vi "Interfaz.vi"() -> ()   [LabVIEW 2018]
uses:
  <vilib>/addons/control/pid/pid.llb/PID EGU to Percentage (DBL).vi
  <vilib>/addons/control/pid/pid.llb/PID Advanced (DBL).vi
  <vilib>/addons/control/pid/NI_PID_pid.lvlib
panel:
  in  "Ring":u16(ring) items=["Principal", "Master", "Slave", "Setting", "Graphics", "Conections"]
  in  "stop":bool
  out "Flux (%)":dbl format="%.2f"
  out "Level (%)":dbl format="%.2f"
  in  "TX Flux":dbl min=0.0 max=0.025
  in  "TX Level":dbl min=0.0 max=0.025
  out "Tab Control":T1(tab)
  out "Level %":dbl
  out "Apertura %":dbl
  out "Flux %":dbl format="%#.1f"
  out "Slide":u8(slide) scale=0.0..100.0
  out "Usuario activo":string
  in  "Please, enterthe  password":string
  in  "Cerrar Sesión":bool
  in  "LSP/ RSP":bool
  out "Fuera De rango":string
  in  "Manual/Auto":bool
  out "Low Limit":bool
  out "High Limit":bool
  in  "Alarm":cluster{dbl, dbl}(slide)={24.183006535947708, 67.3202614379085} scale=0.0..100.0
  in  "SP:":dbl(slide)=54.966887417218544 min=0.0 max=0.0 scale=0.0..100.0
  out "AV:":dbl(slide)=100.0 scale=0.0..100.0
  out "PV:":dbl(slide)=33.01408837398299 scale=0.0..100.0
  in  "MV:":dbl(slide)=100.0 min=0.0 max=100.0 scale=0.0..100.0
  out "RSP:":dbl(slide)=54.966887417218544 min=0.0 max=0.0 scale=0.0..100.0
  out "AV: S":dbl(slide)=100.0 scale=0.0..100.0
  out "Fuera De rango S":string
  in  "Manual/Auto Slave":bool
  out "Low Limit S":bool
  out "High Limit S":bool
  in  "Alarm S":cluster{dbl, dbl}(slide)={24.183006535947708, 67.3202614379085} scale=0.0..100.0
  in  "LSP":dbl(slide)=54.966887417218544 min=0.0 max=0.0 scale=0.0..100.0
  in  "MV: S":dbl(slide)=100.0 scale=-100.0..100.0
  out "PV: S":dbl(slide)=33.01408837398299 scale=0.0..100.0
  in  "setpoint range S":cluster{"setpoint high":dbl, "setpoint low":dbl}={"setpoint high"=100.0, "setpoint low"=0.0} {"setpoint high" min=0.0 max=100.0 format="%.1f"; "setpoint low" min=0.0 max=100.0 format="%.1f"}
  in  "output range S":cluster{"output high":dbl, "output low":dbl}={"output high"=100.0, "output low"=0.0} {"output low" min=0.0 max=100.0 format="%.1f"; "output high" min=0.0 max=100.0 format="%.1f"}
  in  "Inversa/Directa Slave":bool
  in  "PID gains slave":T2={"proportional gain (Kc)"=20.0, "integral time (Ti, min)"=0.008, "derivative time (Td, min)"=0.001} {"derivative time (Td, min)" min=0.0 max=20.0 format="%.2f"; "integral time (Ti, min)" min=0.0 max=50.0 format="%.2f"; "proportional gain (Kc)" min=0.01 max=100.0 format="%.2f"}
  in  "Inversa/Directa":bool
  in  "PID gains":T2={"proportional gain (Kc)"=20.0, "integral time (Ti, min)"=0.008, "derivative time (Td, min)"=0.001} {"derivative time (Td, min)" min=0.0 max=20.0 format="%.2f"; "integral time (Ti, min)" min=0.0 max=50.0 format="%.2f"; "proportional gain (Kc)" min=0.01 max=100.0 format="%.2f"}
  in  "setpoint range":cluster{"setpoint high":dbl, "setpoint low":dbl}={"setpoint high"=100.0, "setpoint low"=0.0} {"setpoint high" min=0.0 max=100.0 format="%.1f"; "setpoint low" min=0.0 max=100.0 format="%.1f"}
  in  "output range":cluster{"output high":dbl, "output low":dbl}={"output high"=100.0, "output low"=0.0} {"output low" min=0.0 max=100.0 format="%.1f"; "output high" min=0.0 max=100.0 format="%.1f"}
  out "Gráfica de Tendencias":T3(graph)
  # "Maestro"
  # "Esclavo"
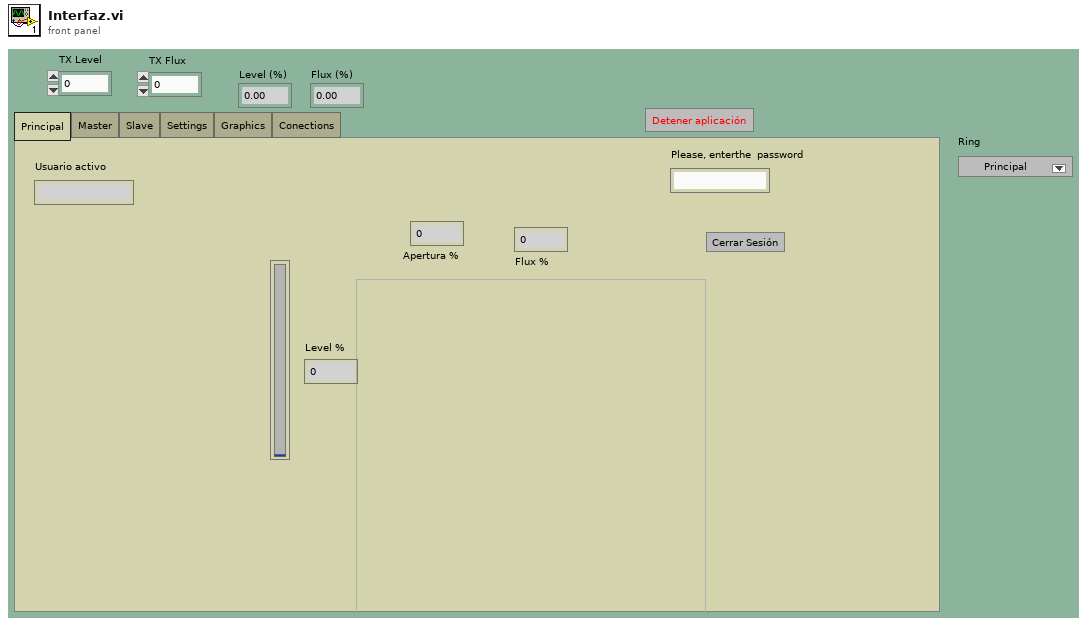
[diagram p1: front panel]
types:
  T1 = enum32{"Principal", "Master", "Slave", "Settings", "Graphics", "Conections"}
  T2 = cluster{"proportional gain (Kc)":dbl, "integral time (Ti, min)":dbl, "derivative time (Td, min)":dbl}
  T3 = cluster{"PV:":dbl, "SP:":dbl, "AV:":dbl, "AV: S":dbl, "PV: S":dbl}
  T4 = cluster{"PV:":dbl, "SP:":dbl, "AV:":dbl, "PV: S":dbl, "AV: S":dbl}
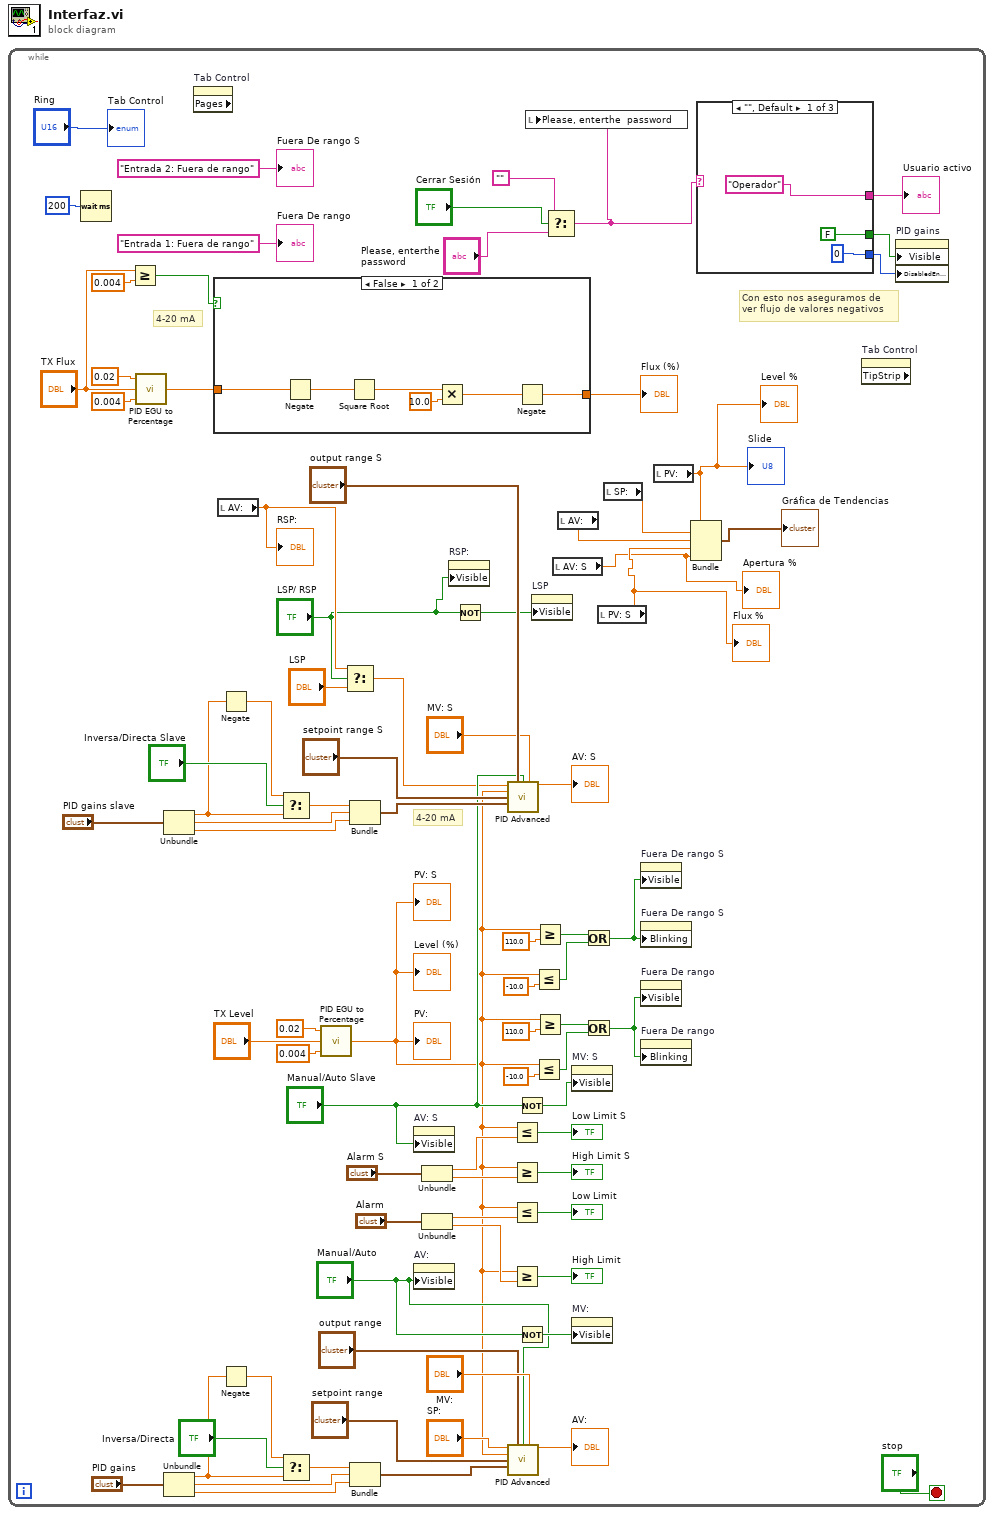
[diagram p0: block diagram]
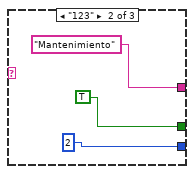
[diagram p2: hidden frame]
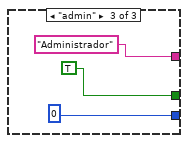
[diagram p3: hidden frame]
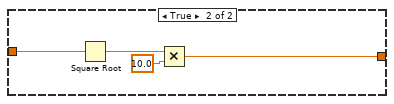
[diagram p4: hidden frame]
diagram:
  n1 = while {
    stop <- "stop" stop-if-true
    # "Con esto nos aseguramos de \nver flujo de valores negativos"
    # "4-20 mA"
    # "4-20 mA"
    n2 = Wait (ms)(milliseconds to wait=u32 200) -> ()  [unwired: 1 out]
    n3 = Greater Or Equal?(x="TX Flux", y=0.004) -> (x >= y?=w75:bool)
    n4 = call-poly <vilib>:"PID EGU to Percentage.vi"("minimum (EGU)"=0.004, "input (EGU)"="TX Flux", "maximum (EGU)"=0.02) -> ("% span"=w74:dbl)
    n5 = Unbundle("PID gains slave") -> ("proportional gain (Kc)"=w41:dbl, "integral time (Ti, min)"=w38:dbl, "derivative time (Td, min)"=w37:dbl)
    n6 = Unbundle("PID gains") -> ("proportional gain (Kc)"=w57:dbl, "integral time (Ti, min)"=w63:dbl, "derivative time (Td, min)"=w62:dbl)
    n7 = property on="Tab Control" class="TabCtl (strict)" props=["Pages"]() -> ()  [unwired: 2 in, 3 out]
    n8 = case shown="False" w75 {
      tunnel: w74 -> [w98 w100]
      tunnel: [w93 w99] -> w73
      frame False {
        n9 = Negate(x=w98) -> (-x=w95:dbl)
        n10 = Square Root(x=w95) -> (sqrt(x)=w97:dbl)
        n11 = Multiply(x=w97, y=10.0) -> (x*y=w94:dbl)
        n12 = Negate(x=w94) -> (-x=w93:dbl)
      }
      frame True {
        n13 = Square Root(x=w100) -> (sqrt(x)=w102:dbl)
        n14 = Multiply(x=w102, y=10.0) -> (x*y=w99:dbl)
      }
    }
    "Flux (%)" <- w73
    n15 = local read "AV:"() -> (w18:dbl)
    "RSP:" <- w18
    n16 = Negate(x=w41) -> (-x=w40:dbl)
    n17 = Negate(x=w57) -> (-x=w58:dbl)
    n18 = Select(t=w40, s="Inversa/Directa Slave", f=w41) -> (s? t:f=w39:dbl)
    n19 = Select(t=w58, s="Inversa/Directa", f=w57) -> (s? t:f=w64:dbl)
    n20 = call-poly <vilib>:"PID EGU to Percentage.vi"("minimum (EGU)"=0.004, "input (EGU)"="TX Level", "maximum (EGU)"=0.02) -> ("% span"=w20:dbl)
    "Level (%)" <- w20
    "PV:" <- w20
    "PV: S" <- w20
    n21 = Select(t=w18, s="LSP/ RSP", f="LSP") -> (s? t:f=w17:dbl)
    n22 = Bundle("proportional gain (Kc)"=w39, "integral time (Ti, min)"=w38, "derivative time (Td, min)"=w37) -> (w36:T2)  [unwired: 1 in]
    n23 = Bundle("proportional gain (Kc)"=w64, "integral time (Ti, min)"=w63, "derivative time (Td, min)"=w62) -> (w61:T2)  [unwired: 1 in]
    n24 = property on="AV: S" class="Slide (strict)"("Visible"="Manual/Auto Slave") -> ()  [unwired: 2 in, 2 out]
    n25 = property on="AV:" class="Slide (strict)"("Visible"="Manual/Auto") -> ()  [unwired: 2 in, 2 out]
    n26 = Unbundle("Alarm S") -> (w30:dbl, w32:dbl)
    n27 = Unbundle("Alarm") -> (w53:dbl, w52:dbl)
    n28 = property on="RSP:" class="Slide (strict)"("Visible"="LSP/ RSP") -> ()  [unwired: 2 in, 2 out]
    n29 = Not(x="LSP/ RSP") -> (.not. x?=w16:bool)
    n30 = call-poly <vilib>:"PID Advanced.vi"("setpoint"=w17, "output range"="output range S", "auto? (T)"="Manual/Auto Slave", "manual control"="MV: S", "process variable"=w20, "setpoint range"="setpoint range S", "PID gains"=w36) -> ("output"=→"AV: S":dbl)  [unwired: 7 in, 1 out]
    n31 = call-poly <vilib>:"PID Advanced.vi"("setpoint"="SP:", "output range"="output range", "auto? (T)"="Manual/Auto", "manual control"="MV:", "process variable"=w20, "setpoint range"="setpoint range", "PID gains"=w61) -> ("output"=→"AV:":dbl)  [unwired: 7 in, 1 out]
    n32 = Less Or Equal?(x=w20, y=w30) -> (x <= y?=→"Low Limit S":bool)
    n33 = Greater Or Equal?(x=w20, y=w32) -> (x >= y?=→"High Limit S":bool)
    n34 = Less Or Equal?(x=w20, y=w53) -> (x <= y?=→"Low Limit":bool)
    n35 = Greater Or Equal?(x=w20, y=w52) -> (x >= y?=→"High Limit":bool)
    n36 = Not(x="Manual/Auto Slave") -> (.not. x?=w34:bool)
    n37 = Not(x="Manual/Auto") -> (.not. x?=w68:bool)
    n38 = property on="LSP" class="Slide (strict)"("Visible"=w16) -> ()  [unwired: 2 in, 2 out]
    n39 = Less Or Equal?(x=w20, y=-10.0) -> (x <= y?=w25:bool)
    n40 = Less Or Equal?(x=w20, y=-10.0) -> (x <= y?=w48:bool)
    n41 = Greater Or Equal?(x=w20, y=110.0) -> (x >= y?=w26:bool)
    n42 = Greater Or Equal?(x=w20, y=110.0) -> (x >= y?=w49:bool)
    n43 = Select(t="", s="Cerrar Sesión", f="Please, enterthe  password") -> (s? t:f=w7:string)
    n44 = local write "Please, enterthe  password"(w7) -> ()
    n45 = local read "AV: S"() -> (w2:dbl)
    "Apertura %" <- w2
    n46 = local read "AV:"() -> (w13:dbl)
    n47 = property on="MV: S" class="Slide (strict)"("Visible"=w34) -> ()  [unwired: 2 in, 2 out]
    n48 = property on="MV:" class="Slide (strict)"("Visible"=w68) -> ()  [unwired: 2 in, 2 out]
    n49 = Or(x=w26, y=w25) -> (x .or. y?=w24:bool)
    n50 = Or(x=w49, y=w48) -> (x .or. y?=w46:bool)
    n51 = local read "PV: S"() -> (w3:dbl)
    "Flux %" <- w3
    n52 = local read "SP:"() -> (w14:dbl)
    n53 = property on="Fuera De rango S" class="Str"("Visible"=w24) -> ()  [unwired: 2 in, 2 out]
    n54 = property on="Fuera De rango S" class="Str"("Blinking"=w24) -> ()  [unwired: 2 in, 2 out]
    n55 = property on="Fuera De rango" class="Str"("Visible"=w46) -> ()  [unwired: 2 in, 2 out]
    n56 = property on="Fuera De rango" class="Str"("Blinking"=w46) -> ()  [unwired: 2 in, 2 out]
    n57 = local read "PV:"() -> (w1:dbl)
    "Slide" <- w1
    "Level %" <- w1
    n58 = Bundle("PV:"=w1, "SP:"=w14, "AV:"=w13, "PV: S"=w3, "AV: S"=w2) -> (→"Gráfica de Tendencias":T4)  [unwired: 1 in]
    n59 = case shown="\"\", Default" w7 {
      tunnel: ["Operador" ("Usuario activo") "Mantenimiento" ("Usuario activo") "Administrador" ("Usuario activo")] -> w11
      tunnel: [FALSE TRUE TRUE] -> w6
      tunnel: [0 2 0] -> w5
      frame "", Default {
      }
      frame "123" {
      }
      frame "admin" {
      }
    }
    "Usuario activo" <- w11
    n60 = property on="Tab Control" class="TabCtl (strict)" props=["TipStrip"]() -> ()  [unwired: 2 in, 3 out]
    n61 = property on="PID gains" class="Clust (strict)"("Visible"=w6, "DisabledEnum"=w5) -> ()  [unwired: 2 in, 2 out]
    "Tab Control" <- "Ring"
    "Fuera De rango" <- "Entrada 1: Fuera de rango" ("Fuera De rango")
    "Fuera De rango S" <- "Entrada 2: Fuera de rango" ("Fuera De rango S")
  }
